vi "SP_Breakdown Summery Yearwise_.vi"() -> ()   [LabVIEW 2017]
uses:
  <vilib>/Math Plots/3D Math Plots/3D Pie/3D Pie XCtrl/3D Pie.xctl
  <vilib>/addons/database/Connection.llb/DB Tools Open Connec (Path).vi
  <vilib>/Math Plots/3D Math Plots/3D Pie/3D Pie Datatype/Public/Plot Helper (Vector).vi
  <vilib>/addons/database/NI_Database_API.lvlib
  <vilib>/Math Plots/3D Math Plots/3D Pie/3D Pie Datatype/3D Pie Datatype.lvclass
panel:
  out "String":string="Processing...\nPlease wait!"
  in  "Cancel Button - Archive":bool
  in  "Get Rport 2":bool
  in  "Download 2":bool
  out "error out":errorcluster
  in  "error in (no error)":errorcluster
  in  "Select Station":string(combo)
  in  "Shift":string(combo)
  out "T":string
  out "P":string
  out "Q":string
  out "M":string
  out "L":string
  out "GL":string
  in  "Select Year":string(combo)
  in  "Select Month":string(combo)
  in  "Tab Control":T1(tab)
  out "Table Control":string[][](table)
  out "heading 6":string="Total"
  out "heading 5":string="Production"
  out "heading 4":string="Qaulity"
  out "heading 3":string="Maintenance"
  out "heading2":string="Logistics"
  out "heading 1":string="Gap Leader"
  out "Count":refnum<class "3D Plot Datatype.lvclass">[](xcontrol)
  out "Duration":refnum<class "3D Plot Datatype.lvclass">[](xcontrol)
  # "Breakdown Summary Report (Year Wise)"
  # "S"
  # "M"
  # "M"
  # "Q"
  # "SS"
  # "TT"
  # "Designed And Developed By - Infinity Automation Systems Pvt. Ltd."
  # "Material"
  # "Safety"
  # "Maintenance"
  # "Quality"
  # "Startup/Setup"
  # "Total"
  # "Month"
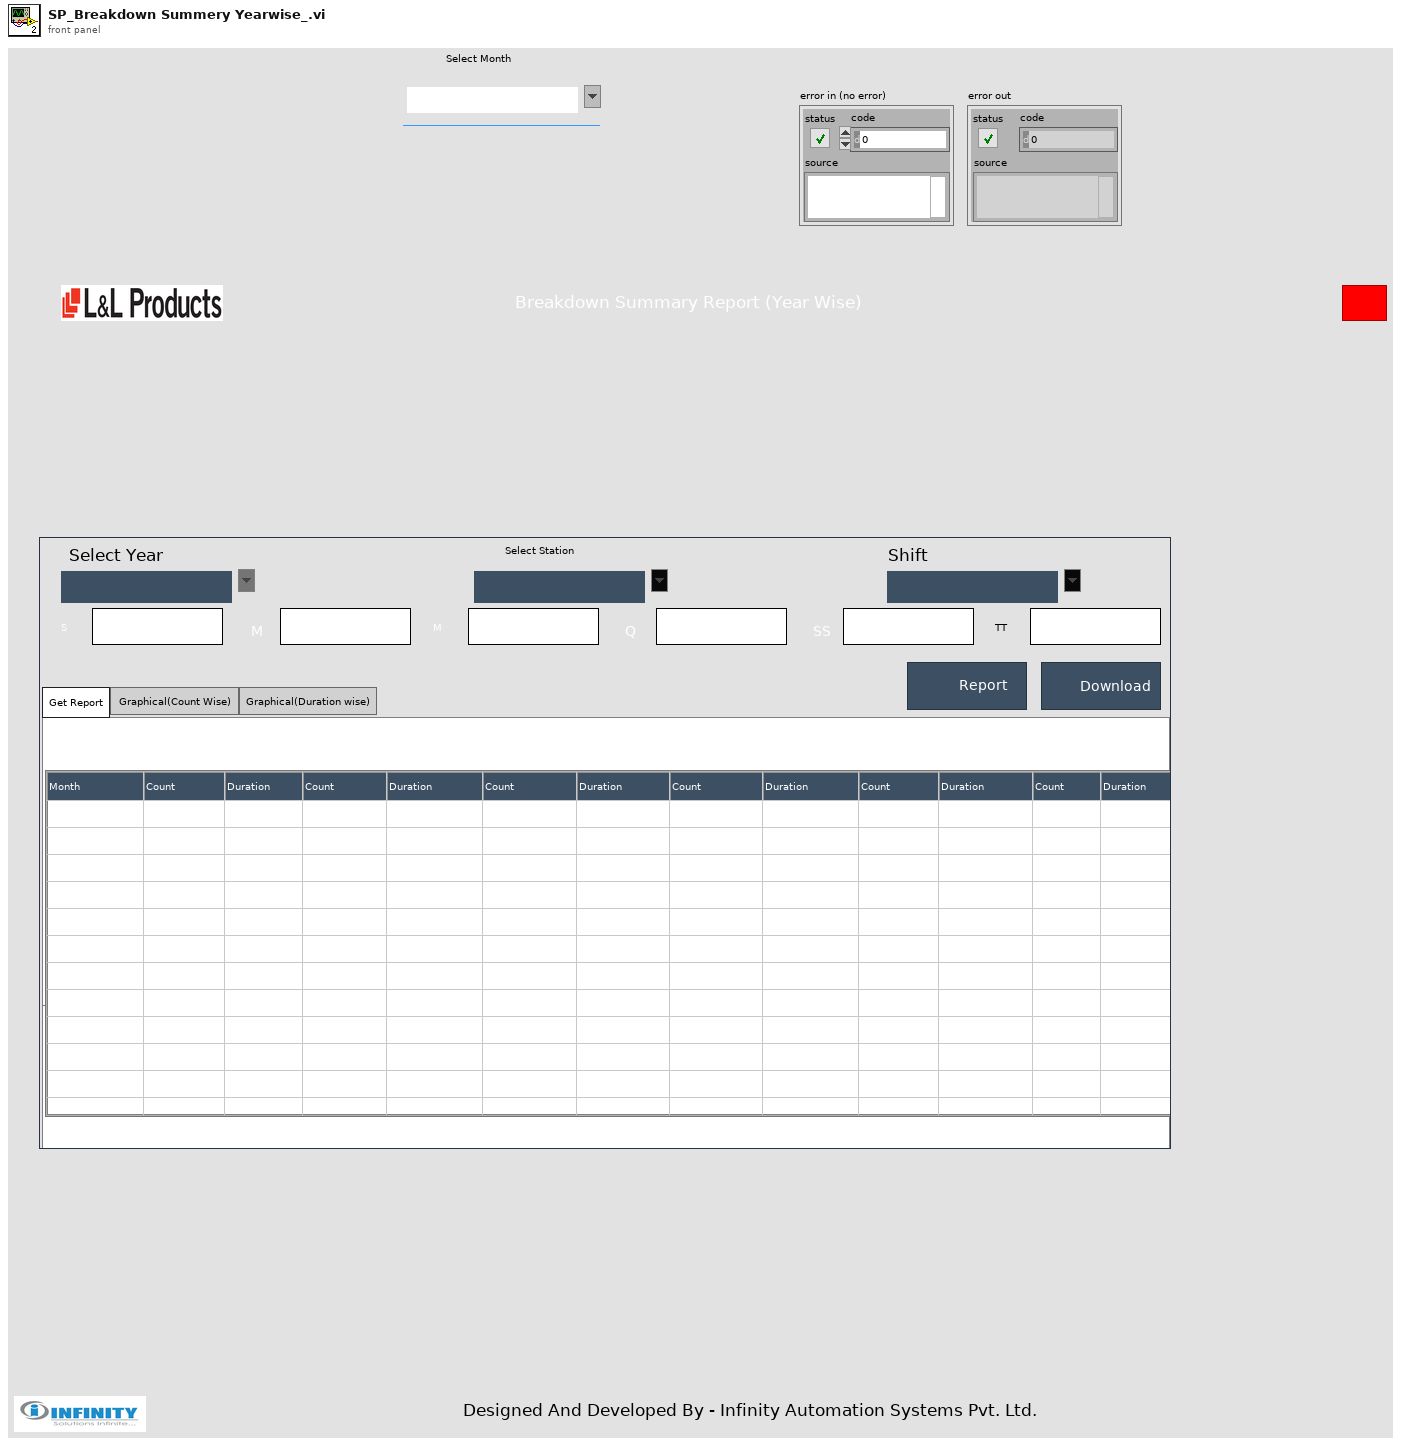
[diagram p1: front panel]
types:
  T1 = enum32{"Get Report", "Graphical(Count Wise) ", "Graphical(Duration wise)"}
  T2 = typedef "NI_Database_API.lvlib/Conn ObjectReference.ctl" = refnum<k1>
  T3 = enum32{"invalid app kind", "Development System", "Run Time System", "Student Edition", "Embedded LabVIEW", "Evaluation", "Custom"}
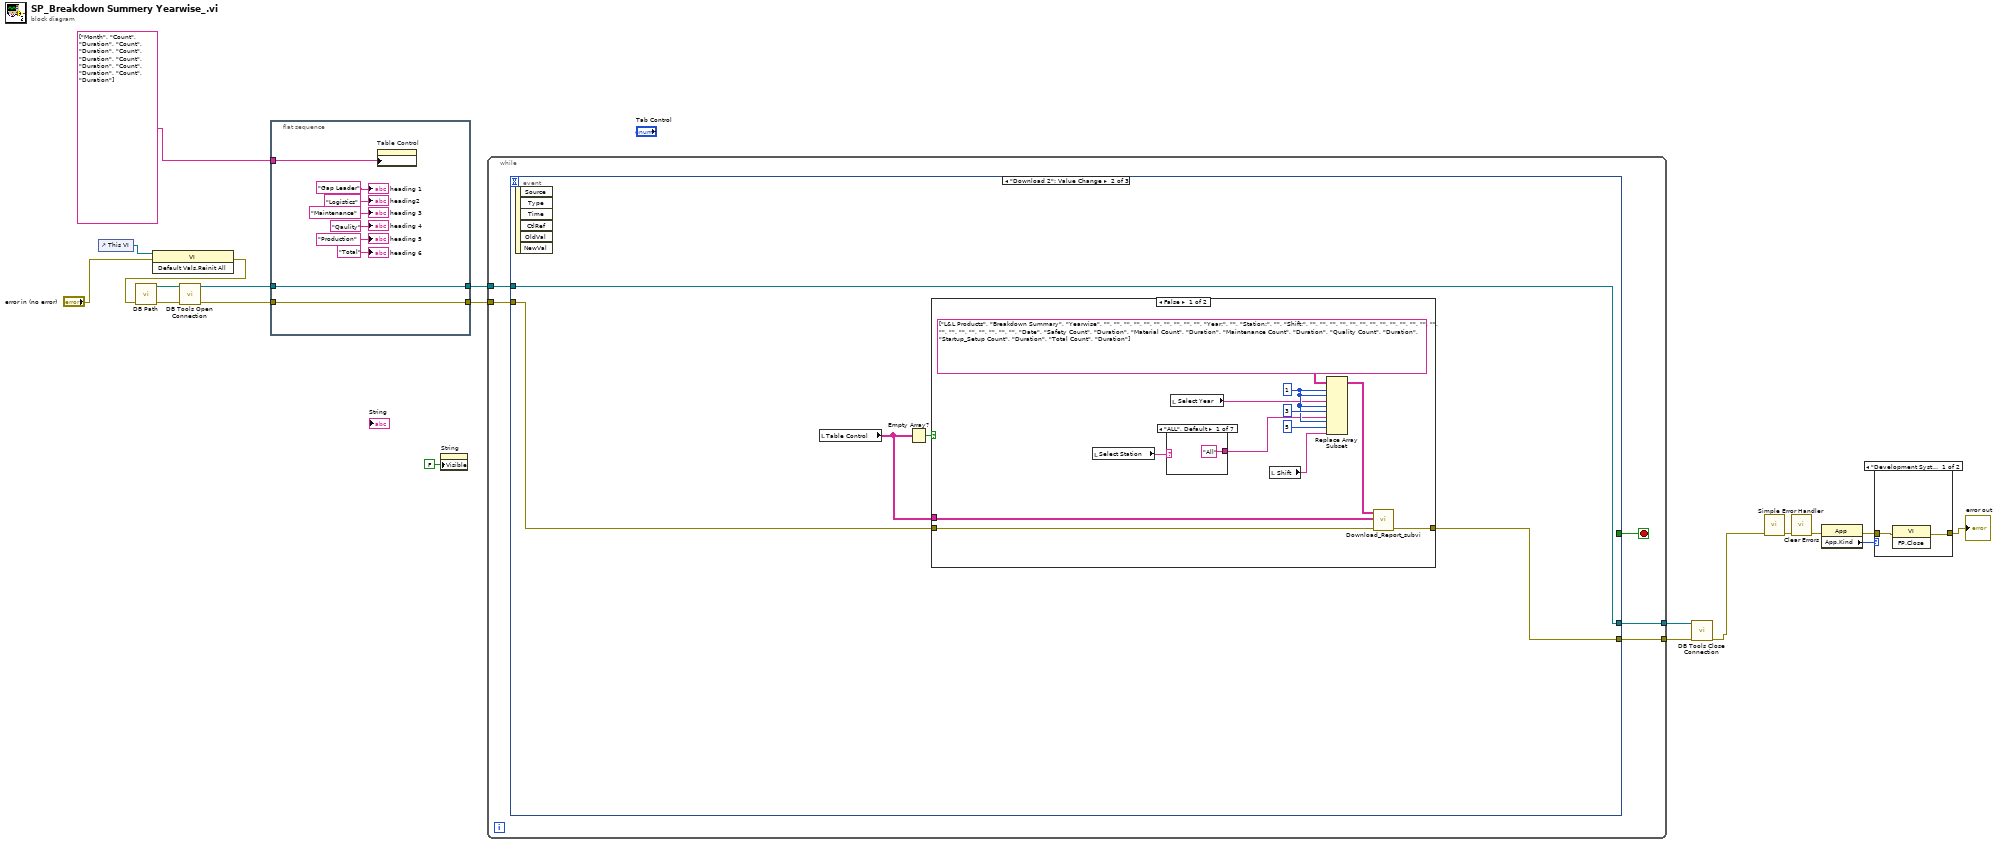
[diagram p0: block diagram]
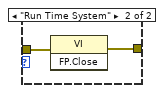
[diagram p2: hidden frame]
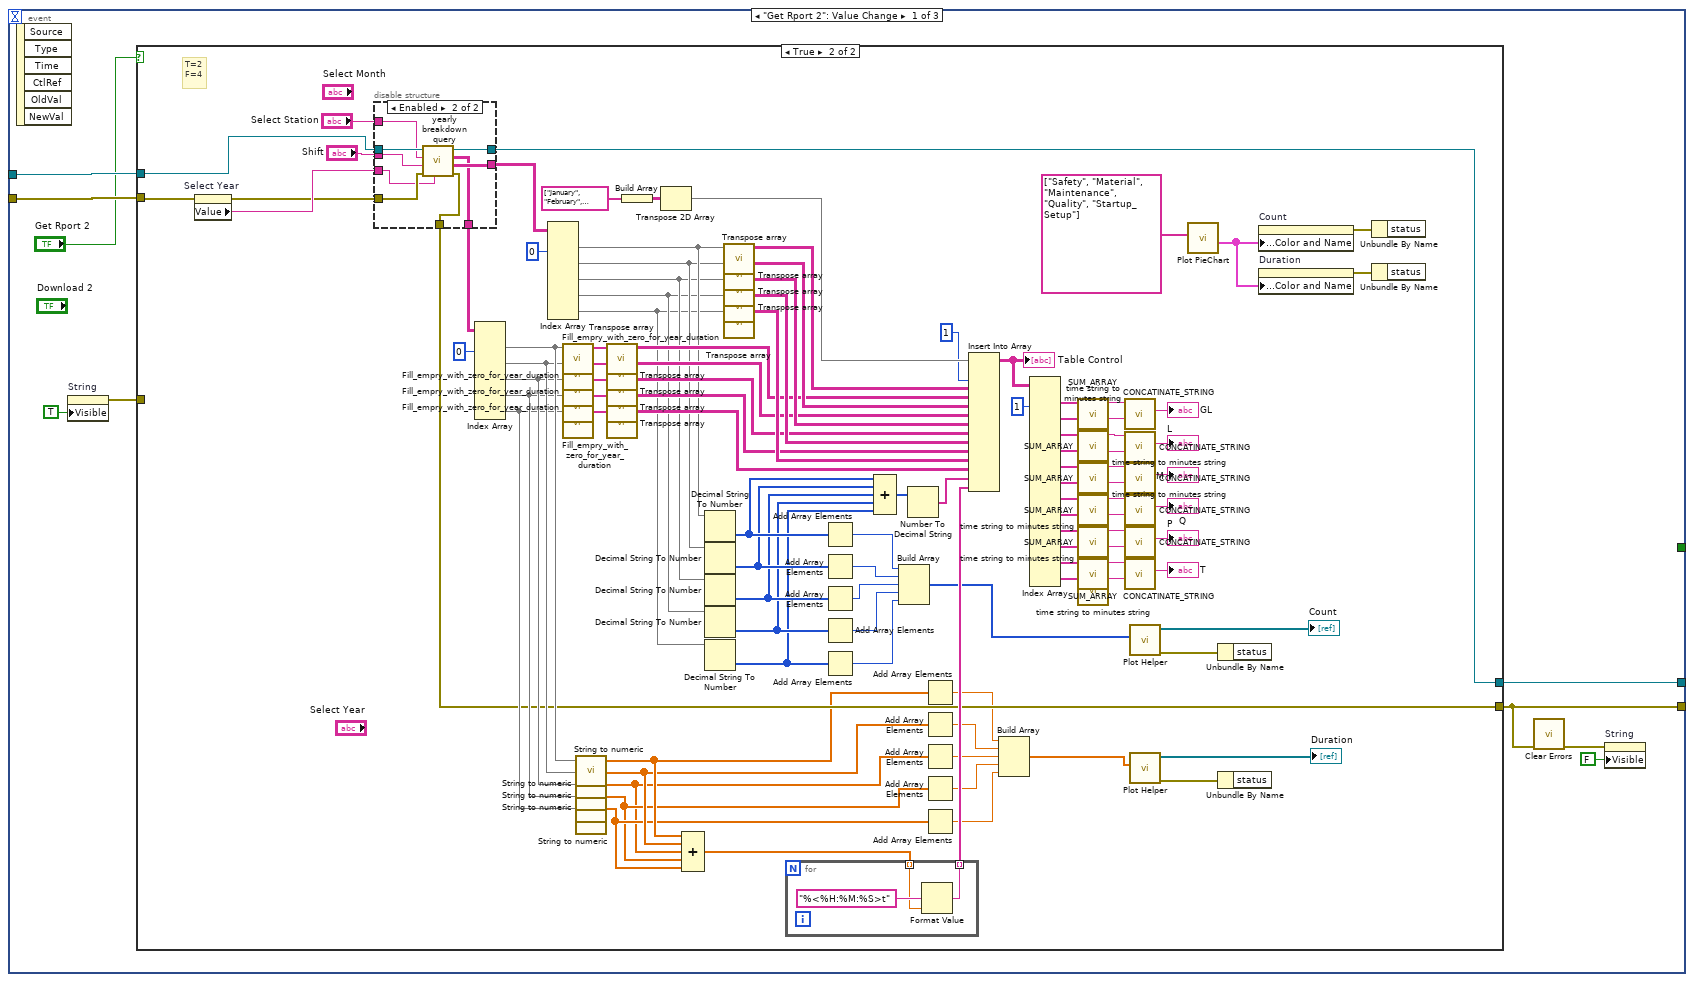
[diagram p3: hidden frame]
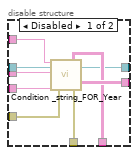
[diagram p5: hidden frame]
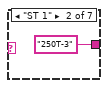
[diagram p6: hidden frame]
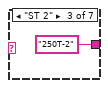
[diagram p7: hidden frame]
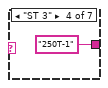
[diagram p8: hidden frame]
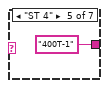
[diagram p9: hidden frame]
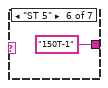
[diagram p10: hidden frame]
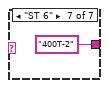
[diagram p11: hidden frame]
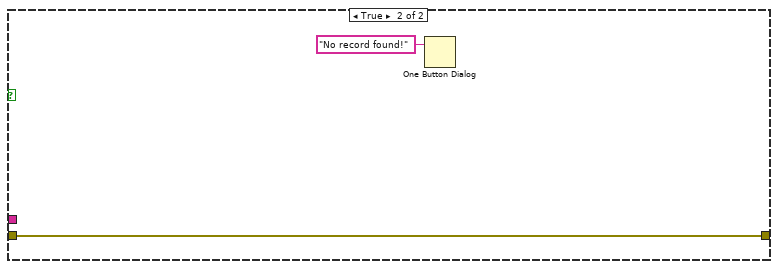
[diagram p12: hidden frame]
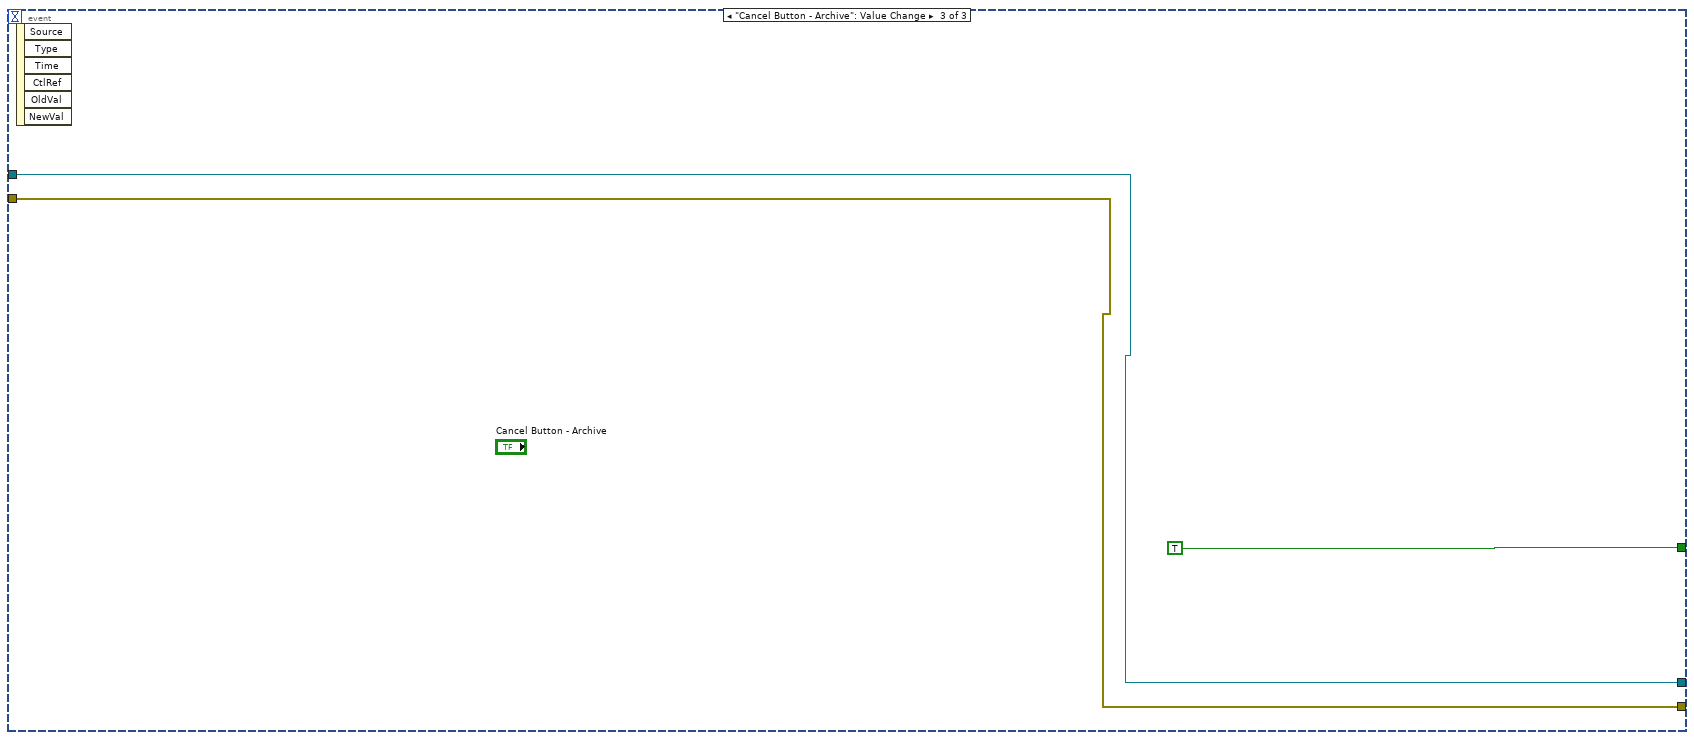
[diagram p13: hidden frame]
diagram:
  n1 = control-ref of="This VI"() -> (w11:refnum<vi>)
  n2 = invoke class="VI" method="Default Vals.Reinit All"(reference=w11, error in="error in (no error)") -> (error out=w9:errorcluster)  [unwired: 1 in, 2 out]
  n3 = call "DB Path.vi"("error in"=w9) -> ("error out"=w19:errorcluster, "DB Path"=w18:path)  [unwired: 9 in]
  n4 = call-poly <vilib>:"DB Tools Open Connection.vi"("error in (no error)"=w19, "connection information"=w18) -> ("error out"=w16:errorcluster, "connection reference"=w15:T2)  [unwired: 6 in]
  n5 = flat-sequence {
    tunnel: [w22] -> w17
    tunnel: w16 -> [w22]
    tunnel: [w21] -> w14
    tunnel: w15 -> [w21]
    tunnel: string[] ["Month", "Count", "Duration", "Count", "Duration", "Count", "Duration", "Count", "Duration", "Count", "Duration", "Count", "Duration"] ("Column Header Strings[]") -> [w20]
    frame #0 {
      n6 = property on="Table Control" class="Tbl (strict)"("Column Headers[]"=w20) -> ()  [unwired: 2 in, 2 out]
      "heading 1" <- "Gap Leader" ("heading 1")
      "heading2" <- "Logistics" ("heading2")
      "heading 3" <- "Maintenance" ("heading 3")
      "heading 4" <- "Qaulity" ("heading 4")
      "heading 5" <- "Production" ("heading 5")
      "heading 6" <- "Total" ("heading 6")
    }
  }
  n7 = property on="String" class="Str"("Visible"=FALSE) -> ()  [unwired: 2 in, 2 out]
  n8 = while {
    tunnel: w17 -> [w32]
    tunnel: w14 -> [w31]
    tunnel: [w30] -> w13
    tunnel: [w29] -> w12
    stop <- w33 stop-if-true
    n9 = event shown="[1] \"Download 2\": Value Change" {
      selector: _ -> [_ _ _]
      dyn-events: _ -> [_ _ _]
      timeout: _ -> [_ _ _]
      tunnel: [_ _ TRUE] -> w33
      tunnel: w32 -> [w42 w177 w199]
      tunnel: w31 -> [w41 w175 w200]
      tunnel: [w35 w176 w199] -> w30
      tunnel: [w40 w175 w200] -> w29
      event "Get Rport 2": Value Change {
        n10 = event-data() -> ()  [unwired: 1 in, 6 out]
        n11 = property on="String" class="Str"("Visible"=TRUE) -> (error out=w37:errorcluster)  [unwired: 2 in, 1 out]
        n12 = case shown="True" "Get Rport 2" {
          tunnel: w42 -> [w43 w151]
          tunnel: w41 -> [w44 w91]
          tunnel: [w43 w75] -> w35
          tunnel: [w44 w90] -> w40
          tunnel: w37 -> [_ _]
          frame False {
          }
          frame True {
            # "T=2\nF=4"
            n13 = property on="Select Year" class="CmbBox"(error in=w151) -> (error out=w92:errorcluster, "Value"=w148:string)  [unwired: 1 in, 1 out]
            n14 = disable-structure shown="Enabled" {
              disable-tunnel: [w160 w165] -> w150
              disable-tunnel: w148 -> [w159 w161]
              disable-tunnel: "Select Station" -> [w158 w163]
              disable-tunnel: "Shift" -> [w157 w162]
              disable-tunnel: [w156 w164] -> w140
              disable-tunnel: w92 -> [w155 w167]
              disable-tunnel: [w154 w166] -> w75
              disable-tunnel: w91 -> [w153 w169]
              disable-tunnel: [w152 w168] -> w90
              frame Disabled {
                n15 = call "Condition _string_FOR_Year.vi"("Select Line 2"=w158, "connection reference"=w153, "Shift"=w157, "year"=w159, "error in (no error)"=w155) -> ("Duration count"=w156:string[][], "error out"=w154:errorcluster, "connection reference 2"=w152:T2, "BD Count"=w160:string[][])  [unwired: 11 in]
              }
              frame Enabled {
                n16 = call "yearly breakdown query.vi"("Year"=w161, "error in"=w167, "Shift"=w162, "Station"=w163, "Refnum in"=w169) -> ("error out"=w166:errorcluster, "Count"=w165:string[][], "Duration"=w164:string[][], "connection reference out"=w168:T2)  [unwired: 3 in]
              }
            }
            n17 = Index Array(array=w140, index (col) #1=0 ("disabled index (col)")) -> (element #1=w118:string[], element #2=w117:string[], element #3=w116:string[], element #4=w115:string[], element #5=w114:string[])  [unwired: 9 in]
            n18 = Index Array(array=w150, index (col) #1=0 ("disabled index (col)")) -> (element #1=w123:string[], element #2=w122:string[], element #3=w121:string[], element #4=w120:string[], element #5=w119:string[])  [unwired: 9 in]
            n19 = call "Fill_empry_with_zero_for_year_duration.vi"("duration In"=w118) -> ("duration out"=w130:string[])  [unwired: 10 in]
            n20 = call "Fill_empry_with_zero_for_year_duration.vi"("duration In"=w117) -> ("duration out"=w129:string[])  [unwired: 10 in]
            n21 = call "Fill_empry_with_zero_for_year_duration.vi"("duration In"=w116) -> ("duration out"=w128:string[])  [unwired: 10 in]
            n22 = call "Fill_empry_with_zero_for_year_duration.vi"("duration In"=w115) -> ("duration out"=w127:string[])  [unwired: 10 in]
            n23 = call "Fill_empry_with_zero_for_year_duration.vi"("duration In"=w114) -> ("duration out"=w126:string[])  [unwired: 10 in]
            n24 = call "String to numeric.vi"("Array"=w118) -> ("Array 2"=w59:dbl[])  [unwired: 4 in]
            n25 = call "String to numeric.vi"("Array"=w117) -> ("Array 2"=w52:dbl[])  [unwired: 4 in]
            n26 = call "String to numeric.vi"("Array"=w116) -> ("Array 2"=w49:dbl[])  [unwired: 4 in]
            n27 = call "String to numeric.vi"("Array"=w115) -> ("Array 2"=w50:dbl[])  [unwired: 4 in]
            n28 = call "String to numeric.vi"("Array"=w114) -> ("Array 2"=w51:dbl[])  [unwired: 4 in]
            n29 = call "Transpose array.vi"("BD Count"=w130) -> ("Array"=w125:string[][])  [unwired: 10 in]
            n30 = call "Transpose array.vi"("BD Count"=w129) -> ("Array"=w135:string[][])  [unwired: 10 in]
            n31 = call "Transpose array.vi"("BD Count"=w128) -> ("Array"=w134:string[][])  [unwired: 10 in]
            n32 = call "Transpose array.vi"("BD Count"=w127) -> ("Array"=w133:string[][])  [unwired: 10 in]
            n33 = call "Transpose array.vi"("BD Count"=w126) -> ("Array"=w132:string[][])  [unwired: 10 in]
            n34 = Build Array(string[] ["January", "February", "March", "April", "May", "June", "July", "August", "September", "October", "November", "December"]) -> (w145:string[][])
            n35 = Transpose 2D Array(2D array=w145) -> (transposed array=w144:string[][])
            n36 = Compound Arithmetic op=ADD(w59, w52, w49, w50, w51) -> (w89:dbl[])
            n37 = Decimal String To Number(string=w123) -> (number=w58:i32[])  [unwired: 2 in, 1 out]
            n38 = Decimal String To Number(string=w122) -> (number=w57:i32[])  [unwired: 2 in, 1 out]
            n39 = Decimal String To Number(string=w121) -> (number=w56:i32[])  [unwired: 2 in, 1 out]
            n40 = Decimal String To Number(string=w120) -> (number=w55:i32[])  [unwired: 2 in, 1 out]
            n41 = Decimal String To Number(string=w119) -> (number=w54:i32[])  [unwired: 2 in, 1 out]
            n42 = call "Transpose array.vi"("BD Count"=w123) -> ("Array"=w143:string[][])  [unwired: 10 in]
            n43 = call "Transpose array.vi"("BD Count"=w122) -> ("Array"=w139:string[][])  [unwired: 10 in]
            n44 = call "Transpose array.vi"("BD Count"=w121) -> ("Array"=w138:string[][])  [unwired: 10 in]
            n45 = call "Transpose array.vi"("BD Count"=w120) -> ("Array"=w137:string[][])  [unwired: 10 in]
            n46 = call "Transpose array.vi"("BD Count"=w119) -> ("Array"=w136:string[][])  [unwired: 10 in]
            n47 = for {
              tunnel: w89 -> [w171] mode=indexing
              tunnel: [w170] -> w88 mode=indexing
              n48 = Format Value(format string="%<%H:%M:%S>t", value (0)=w171) -> (output string=w170:string)  [unwired: 1 in]
            }
            n49 = Add Array Elements(numeric array=w58) -> (sum=w70:i32)
            n50 = Add Array Elements(numeric array=w57) -> (sum=w69:i32)
            n51 = Add Array Elements(numeric array=w56) -> (sum=w68:i32)
            n52 = Add Array Elements(numeric array=w55) -> (sum=w67:i32)
            n53 = Add Array Elements(numeric array=w54) -> (sum=w66:i32)
            n54 = Compound Arithmetic op=ADD(w58, w57, w56, w55, w54) -> (w124:i32[])
            n55 = Build Array(w70, w69, w68, w67, w66) -> (w53:i32[])
            n56 = Number To Decimal String(number=w124) -> (decimal integer string=w93:string[])  [unwired: 1 in]
            n57 = Add Array Elements(numeric array=w59) -> (sum=w61:dbl)
            n58 = Add Array Elements(numeric array=w52) -> (sum=w62:dbl)
            n59 = Add Array Elements(numeric array=w49) -> (sum=w63:dbl)
            n60 = Add Array Elements(numeric array=w50) -> (sum=w64:dbl)
            n61 = Add Array Elements(numeric array=w51) -> (sum=w65:dbl)
            n62 = Insert Into Array(array=w144, index (col)=1 ("index"), new element #1=w143, new element #2=w125, new element #3=w139, new element #4=w135, new element #5=w138, new element #6=w134, new element #7=w137, new element #8=w133, new element #9=w136, new element #10=w132, new element #11=w93, new element #12=w88) -> (w100:string[][])  [unwired: 1 in]
            "Table Control" <- w100
            n63 = Build Array(w61, w62, w63, w64, w65) -> (w60:dbl[])
            n64 = Index Array(array=w100, index (col) #1=1 ("disabled index (col)")) -> (element #1=w112:string[], element #2=w82:string[], element #3=w111:string[], element #4=w81:string[], element #5=w110:string[], element #6=w79:string[], element #7=w109:string[], element #8=w78:string[], element #9=w108:string[], element #10=w77:string[], element #11=w107:string[], element #12=w87:string[])  [unwired: 23 in]
            n65 = call "SUM_ARRAY.vi"("Array"=w112) -> ("F-format string"=w106:string)  [unwired: 6 in]
            n66 = call "time string to minutes string.vi"("Array"=w82) -> ("output string"=w83:string)  [unwired: 10 in]
            n67 = call "SUM_ARRAY.vi"("Array"=w111) -> ("F-format string"=w105:string)  [unwired: 6 in]
            n68 = call "time string to minutes string.vi"("Array"=w81) -> ("output string"=w80:string)  [unwired: 10 in]
            n69 = call "SUM_ARRAY.vi"("Array"=w110) -> ("F-format string"=w104:string)  [unwired: 6 in]
            n70 = call "time string to minutes string.vi"("Array"=w79) -> ("output string"=w84:string)  [unwired: 10 in]
            n71 = call "SUM_ARRAY.vi"("Array"=w109) -> ("F-format string"=w103:string)  [unwired: 6 in]
            n72 = call "time string to minutes string.vi"("Array"=w78) -> ("output string"=w85:string)  [unwired: 10 in]
            n73 = call "SUM_ARRAY.vi"("Array"=w108) -> ("F-format string"=w102:string)  [unwired: 6 in]
            n74 = call "time string to minutes string.vi"("Array"=w77) -> ("output string"=w76:string)  [unwired: 10 in]
            n75 = call "SUM_ARRAY.vi"("Array"=w107) -> ("F-format string"=w101:string)  [unwired: 6 in]
            n76 = call "time string to minutes string.vi"("Array"=w87) -> ("output string"=w86:string)  [unwired: 10 in]
            n77 = call "CONCATINATE_STRING.vi"("F-format string"=w83, "F-format string 2"=w106) -> ("concatenated string"=→"GL":string)  [unwired: 9 in]
            n78 = call "CONCATINATE_STRING.vi"("F-format string"=w80, "F-format string 2"=w105) -> ("concatenated string"=→"L":string)  [unwired: 9 in]
            n79 = call "CONCATINATE_STRING.vi"("F-format string"=w84, "F-format string 2"=w104) -> ("concatenated string"=→"M":string)  [unwired: 9 in]
            n80 = call "CONCATINATE_STRING.vi"("F-format string"=w85, "F-format string 2"=w103) -> ("concatenated string"=→"Q":string)  [unwired: 9 in]
            n81 = call "CONCATINATE_STRING.vi"("F-format string"=w76, "F-format string 2"=w102) -> ("concatenated string"=→"P":string)  [unwired: 9 in]
            n82 = call "CONCATINATE_STRING.vi"("F-format string"=w86, "F-format string 2"=w101) -> ("concatenated string"=→"T":string)  [unwired: 9 in]
            n83 = call-poly <vilib>:"Plot Helper.vi"("x vector"=w53) -> ("error out"=w74:errorcluster, "3D Plot lvclass Array out"=→"Count":refnum<class "3D Plot Datatype.lvclass">[])  [unwired: 2 in, 7 out]
            n84 = call-poly <vilib>:"Plot Helper.vi"("x vector"=w60) -> ("error out"=w73:errorcluster, "3D Plot lvclass Array out"=→"Duration":refnum<class "3D Plot Datatype.lvclass">[])  [unwired: 2 in, 7 out]
            n85 = call "Plot PieChart.vi"("Label"=string[] ["Safety", "Material", "Maintenance", "Quality", "Startup_Setup"]) -> ("Labelling"=w45:cluster{dbl, "String":string}[])  [unwired: 10 in]
            n86 = Unbundle By Name(w74) -> ()  [unwired: 1 out]
            n87 = Unbundle By Name(w73) -> ()  [unwired: 1 out]
            n88 = property on="Count" class="3D Pie (strict)"("Plot Specific:Color and Name"=w45) -> (error out=w47:errorcluster)  [unwired: 2 in, 1 out]
            n89 = property on="Duration" class="3D Pie (strict)"("Plot Specific:Color and Name"=w45) -> (error out=w46:errorcluster)  [unwired: 2 in, 1 out]
            n90 = Unbundle By Name(w47) -> ()  [unwired: 1 out]
            n91 = Unbundle By Name(w46) -> ()  [unwired: 1 out]
          }
        }
        n92 = call <vilib>:"Clear Errors.vi"("error in (no error)"=w35) -> ("error out"=w34:errorcluster)  [unwired: 5 in, 1 out]
        n93 = property on="String" class="Str"(error in=w34, "Visible"=FALSE) -> ()  [unwired: 1 in, 2 out]
      }
      event "Download 2": Value Change {
        n94 = event-data() -> ()  [unwired: 1 in, 6 out]
        n95 = local read "Table Control"() -> (w173:string[][])
        n96 = Empty Array?(array=w173) -> (empty?=w174:bool)
        n97 = case shown="False" w174 {
          tunnel: w177 -> [w189 w198]
          tunnel: w173 -> [w188 _]
          tunnel: [w187 w198] -> w176
          frame False {
            w183 = 1 ("index (row)")
            n98 = local read "Select Station"() -> (w179:string)
            n99 = case shown="\"ALL\", Default" w179 {
              tunnel: ["All" "250T-3" "250T-2" "250T-1" "400T-1" "150T-1" "400T-2"] -> w180
              frame "ALL", Default {
              }
              frame "ST 1" {
              }
              frame "ST 2" {
              }
              frame "ST 3" {
              }
              frame "ST 4" {
              }
              frame "ST 5" {
              }
              frame "ST 6" {
              }
            }
            n100 = local read "Select Year"() -> (w181:string)
            n101 = local read "Shift"() -> (w178:string)
            n102 = Replace Array Subset(array=string[][] [["L&L Products", "Breakdown Summary", "Yearwise", "", "", "", "", "", "", "", "", "", ""], ["Year:", "", "Station:", "", "Shift:", "", "", "", "", "", "", "", ""], ["", "", "", "", "", "", "", "", "", "", "", "", ""], ["Date", "Safety Count", "Duration", "Material Count", "Duration", "Maintenance Count", "Duration", "Quality Count", "Duration", "Startup_Setup Count", "Duration", "Total Count", "Duration"]] ("Column Header Strings[]"), new element #1=w181, index (row) #1=w183, index (col) #1=w183, new element #2=w180, index (row) #2=w183, index (col) #2=3 ("disabled index (col)"), new element #3=w178, index (row) #3=w183, index (col) #3=5 ("disabled index (col)")) -> (w182:string[][])
            n103 = call "Download_Report_subvi.vi"("error in (no error)"=w189, "Value"=w188, "Column Header Strings[]"=w182) -> ("error out"=w187:errorcluster)  [unwired: 8 in]
          }
          frame True {
            n104 = One Button Dialog(message="No record found!") -> ()  [unwired: 1 in, 1 out]
          }
        }
      }
      event "Cancel Button - Archive": Value Change {
        n105 = event-data() -> ()  [unwired: 1 in, 6 out]
      }
    }
  }
  n106 = call <vilib>:"DB Tools Close Connection.vi"("error in (no error)"=w13, "connection reference"=w12) -> ("error out"=w4:errorcluster)  [unwired: 5 in]
  n107 = call <vilib>:"Simple Error Handler.vi"("error in (no error)"=w4) -> ("error out"=w8:errorcluster)  [unwired: 4 in, 4 out]
  n108 = call <vilib>:"Clear Errors.vi"("error in (no error)"=w8) -> ("error out"=w7:errorcluster)  [unwired: 5 in, 1 out]
  n109 = property class="App"(error in=w7) -> (error out=w6:errorcluster, "App.Kind"=w5:T3)  [unwired: 1 in, 1 out]
  n110 = case shown="\"Development System\", Default" w5 {
    tunnel: w6 -> [w203 w205]
    tunnel: [w202 w204] -> w3
    frame "Development System", Default {
      n111 = invoke class="VI" method="FP.Close"(error in=w203) -> (error out=w202:errorcluster)  [unwired: 2 in, 2 out]
    }
    frame "Run Time System" {
      n112 = invoke class="VI" method="FP.Close"(error in=w205) -> (error out=w204:errorcluster)  [unwired: 2 in, 2 out]
    }
  }
  "error out" <- w3
